vi "Assert.vi"(4 "Variable Y":variant, 6 "Variable X":variant, 11 "Assert in":refnum<class "Assert.lvclass">) -> (2 "Assert?":bool)   [LabVIEW 2017, in "Run Time Assertions.lvlib" / "Assert.lvclass"]
uses:
  <vilib>/gpm_packages/@cs/run-time-assertions/Source/Assert/Assert.lvclass
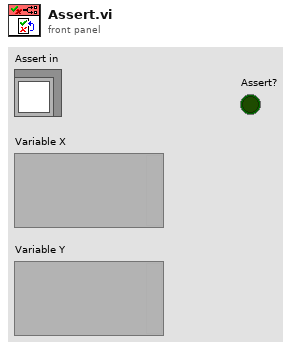
[diagram p1: front panel]
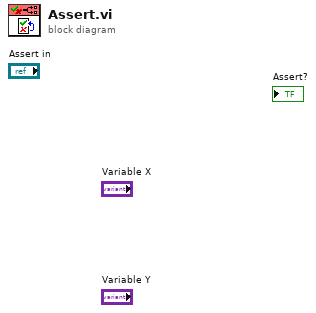
[diagram p0: block diagram]
diagram:
